vi "Table Control_2D.vi"(0 "CtlRef":refnum<vi>, 5 "CharIn":i16, 7 "VKey":T1, 9 "ScanCode":i16) -> (6 "CharOut":i16, 15 "Discard?":bool)   [LabVIEW 2013]
uses:
  <vilib>/Utility/miscctls.llb/LVRowAndColumnTypeDef.ctl
  <vilib>/event_ctls.llb/eventvkey.ctl
panel:
  in  "Header Row(F)/Column(T)":bool
  in  "Valid Indexes":i32[](array[numeric])
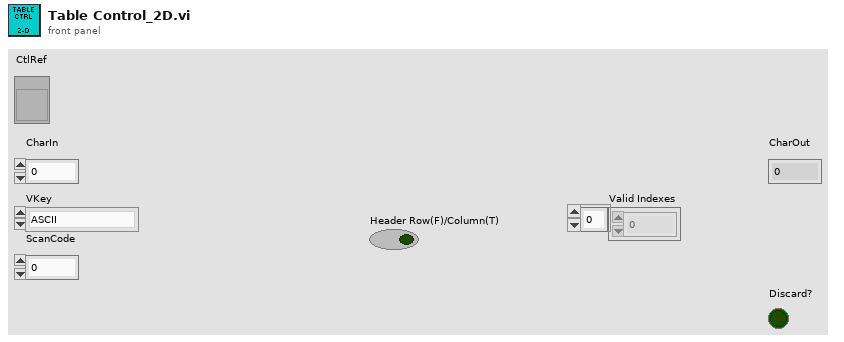
[diagram p1: front panel]
types:
  T1 = typedef "eventvkey.ctl" = enum16{"ASCII", "Enter", "Return", "Shift", "Ctrl", "Alt", "Cmd", "Opt", "Caps", "NumLock", "Clear", "Break", "Up", "Down", "Left", "Right", "Insert", "Delete", "Home", "End", "PageUp", "PageDown", "Escape", "Help", "Pause", "ScrollLock", "F1", "F2", "F3", "F4", "F5", "F6", "F7", "F8", "F9", "F10", "F11", "F12", "F13", "F14", "F15", "F16", "F17", "F18", "F19", "F20", "F21", "F22", "F23", "F24", "Play", "VolumeUp", "VolumeDown", "Mute", "Two Byte Char"}
  T2 = typedef "LVRowAndColumnTypeDef.ctl" = cluster{"Row":i32, "Column":i32}
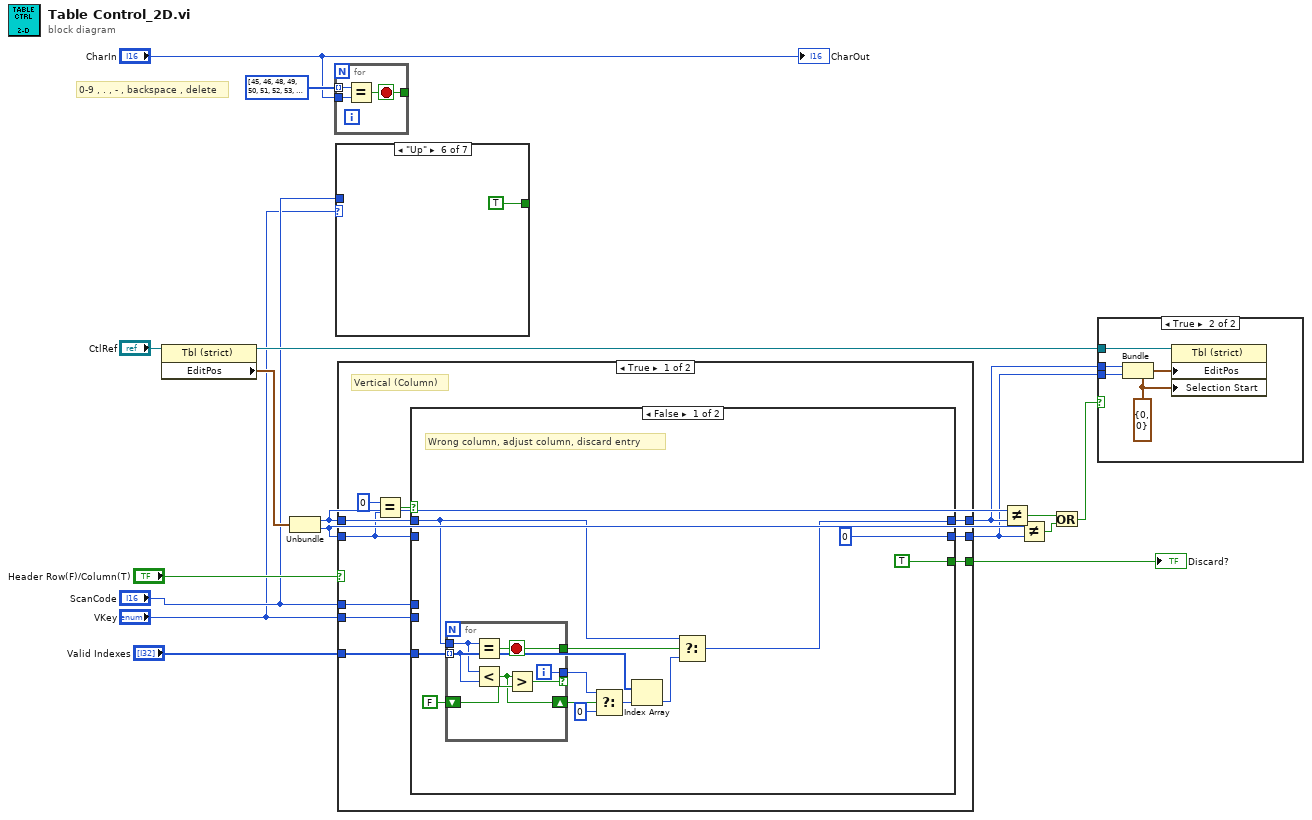
[diagram p0: block diagram]
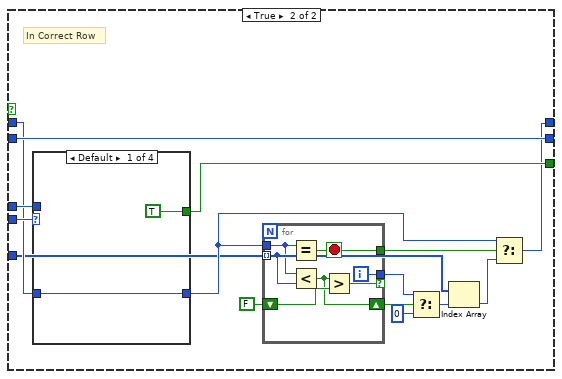
[diagram p3: hidden frame]
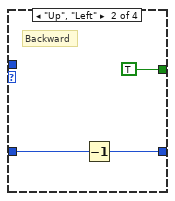
[diagram p4: hidden frame]
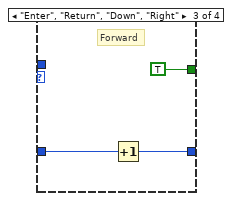
[diagram p5: hidden frame]
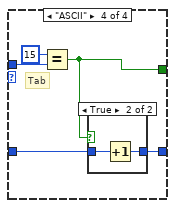
[diagram p6: hidden frame]
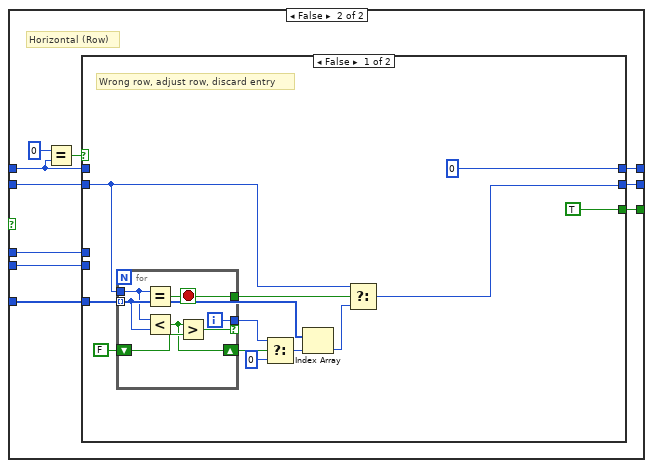
[diagram p8: hidden frame]
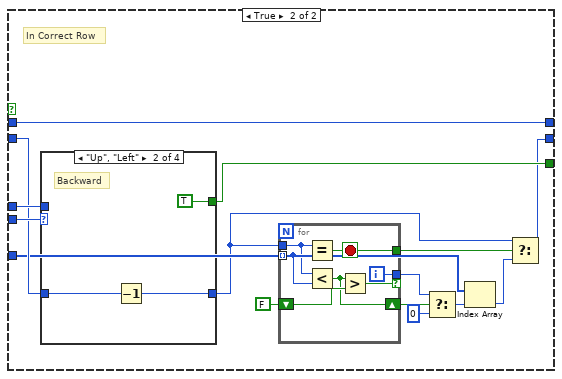
[diagram p9: hidden frame]
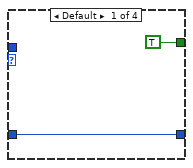
[diagram p10: hidden frame]
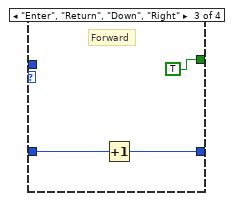
[diagram p11: hidden frame]
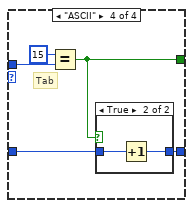
[diagram p12: hidden frame]
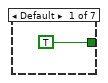
[diagram p14: hidden frame]
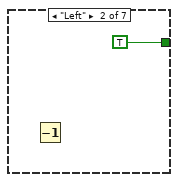
[diagram p15: hidden frame]
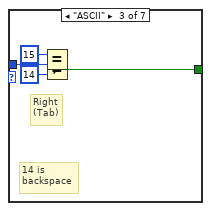
[diagram p16: hidden frame]
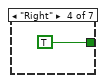
[diagram p17: hidden frame]
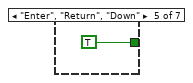
[diagram p18: hidden frame]
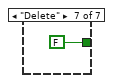
[diagram p19: hidden frame]
diagram:
  # "0-9 , . , - , backspace , delete"
  n1 = property on="Property Node" class="Tbl (strict)"(reference="CtlRef") -> (reference out=w4:refnum<vi>, "EditPos"=w5:T2)  [unwired: 1 in, 1 out]
  n2 = Unbundle(w5) -> ("Row"=w11:i32, "Column"=w9:i32)
  n3 = for {
    tunnel: i16[] [45, 46, 48, 49, 50, 51, 52, 53, 54, 55, 56, 57] -> [w20] mode=indexing
    tunnel: "CharIn" -> [w19]
    tunnel: [w18] -> _
    stop <- w18 stop-if-true
    n4 = Equal?(x=w20, y=w19) -> (x = y?=w18:bool)
  }
  n5 = case shown="\"Up\"" "VKey" {
    tunnel: "ScanCode" -> [_ _ w27 _ _ _ _]
    tunnel: [TRUE TRUE w25 TRUE TRUE TRUE FALSE] -> _
    frame Default {
    }
    frame "Left" {
      n6 = Decrement() -> (x=w24:dbl, x-1=w23:dbl)
    }
    frame "ASCII" {
      # "14 is\nbackspace"
      # "Right\n(Tab)"
      n7 = Equal?(x=i16 15, y=w27) -> ()  [unwired: 1 out]
      n8 = Not Equal?(x=w27, y=i16 14 ("x")) -> (x != y?=w25:bool)
    }
    frame "Right" {
    }
    frame "Enter", "Return", "Down" {
    }
    frame "Up" {
    }
    frame "Delete" {
    }
  }
  n9 = case shown="True" "Header Row(F)/Column(T)" {
    tunnel: w11 -> [w42 w103]
    tunnel: w9 -> [w34 w107]
    tunnel: "Valid Indexes" -> [w36 w106]
    tunnel: [w41 w105] -> w10
    tunnel: [w40 w104] -> w8
    tunnel: [w39 w102] -> w1
    tunnel: "ScanCode" -> [w38 w101]
    tunnel: "VKey" -> [w37 w100]
    frame True {
      # "Vertical (Column)"
      n10 = Equal?(x=0, y=w34) -> (x = y?=w33:bool)
      n11 = case shown="False" w33 {
        tunnel: w34 -> [_ w73]
        tunnel: w36 -> [w48 w62]
        tunnel: [w44 w63] -> w41
        tunnel: [0 w73] -> w40
        tunnel: w42 -> [w45 w72]
        tunnel: [TRUE w74] -> w39
        tunnel: w38 -> [_ w76]
        tunnel: w37 -> [_ w75]
        frame False {
          # "Wrong column, adjust column, discard entry"
          n12 = for {
            tunnel: w48 -> [w59] mode=indexing
            tunnel: w45 -> [w60]
            tunnel: [w61] -> w54
            shift-right: [w55] -> w52
            shift-left: FALSE -> [w58]
            tunnel: [w57] -> w51 if=w56
            i -> [w57]
            stop <- w61 stop-if-true
            n13 = Equal?(x=w60, y=w59) -> (x = y?=w61:bool)
            n14 = Less?(x=w60, y=w59) -> (x < y?=w55:bool)
            n15 = Greater?(x=w55, y=w58) -> (0:w56:bool)
          }
          n16 = Select(t=w51, s=w52, f=0) -> (s? t:f=w49:i32)
          n17 = Index Array(array=w48, index=w49) -> (element=w47:i32)
          n18 = Select(t=w45, s=w54, f=w47) -> (s? t:f=w44:i32)
        }
        frame True {
          # "In Correct Row"
          n19 = case shown="Default" w75 {
            tunnel: w76 -> [_ _ _ w95]
            tunnel: w72 -> [w85 w87 w90 w94]
            tunnel: [w85 w86 w89 w93] -> w64
            tunnel: [TRUE TRUE TRUE w92] -> w74
            frame Default {
            }
            frame "Up", "Left" {
              # "Backward"
              n20 = Decrement(x=w87) -> (x-1=w86:i32)
            }
            frame "Enter", "Return", "Down", "Right" {
              # "Forward"
              n21 = Increment(x=w90) -> (x+1=w89:i32)
            }
            frame "ASCII" {
              # "Tab"
              n22 = Equal?(x=i16 15, y=w95) -> (x = y?=w92:bool)
              n23 = case shown="True" w92 {
                tunnel: w94 -> [w97 w99]
                tunnel: [w97 w98] -> w93
                frame False {
                }
                frame True {
                  n24 = Increment(x=w99) -> (x+1=w98:i32)
                }
              }
            }
          }
          n25 = for {
            tunnel: w62 -> [w81] mode=indexing
            tunnel: w64 -> [w82]
            tunnel: [w83] -> w71
            shift-right: [w77] -> w69
            shift-left: FALSE -> [w80]
            tunnel: [w79] -> w68 if=w78
            i -> [w79]
            stop <- w83 stop-if-true
            n26 = Equal?(x=w82, y=w81) -> (x = y?=w83:bool)
            n27 = Less?(x=w82, y=w81) -> (x < y?=w77:bool)
            n28 = Greater?(x=w77, y=w80) -> (0:w78:bool)
          }
          n29 = Select(t=w68, s=w69, f=0) -> (s? t:f=w66:i32)
          n30 = Index Array(array=w62, index=w66) -> (element=w65:i32)
          n31 = Select(t=w64, s=w71, f=w65) -> (s? t:f=w63:i32)
        }
      }
    }
    frame False {
      # "Horizontal (Row)"
      n32 = Equal?(x=0, y=w103) -> (x = y?=w108:bool)
      n33 = case shown="False" w108 {
        tunnel: w107 -> [w112 w140]
        tunnel: w106 -> [w114 w130]
        tunnel: [0 w143] -> w105
        tunnel: [w111 w131] -> w104
        tunnel: w103 -> [_ w143]
        tunnel: [TRUE w139] -> w102
        tunnel: w101 -> [_ w142]
        tunnel: w100 -> [_ w141]
        frame False {
          # "Wrong row, adjust row, discard entry"
          n34 = for {
            tunnel: w114 -> [w126] mode=indexing
            tunnel: w112 -> [w127]
            tunnel: [w128] -> w120
            shift-right: [w122] -> w118
            shift-left: FALSE -> [w125]
            tunnel: [w124] -> w117 if=w123
            i -> [w124]
            stop <- w128 stop-if-true
            n35 = Equal?(x=w127, y=w126) -> (x = y?=w128:bool)
            n36 = Less?(x=w127, y=w126) -> (x < y?=w122:bool)
            n37 = Greater?(x=w122, y=w125) -> (0:w123:bool)
          }
          n38 = Select(t=w117, s=w118, f=0) -> (s? t:f=w115:i32)
          n39 = Index Array(array=w114, index=w115) -> (element=w113:i32)
          n40 = Select(t=w112, s=w120, f=w113) -> (s? t:f=w111:i32)
        }
        frame True {
          # "In Correct Row"
          n41 = case shown="\"Up\", \"Left\"" w141 {
            tunnel: w142 -> [_ _ _ w162]
            tunnel: w140 -> [w152 w154 w157 w161]
            tunnel: [w152 w153 w156 w160] -> w129
            tunnel: [TRUE TRUE TRUE w159] -> w139
            frame Default {
            }
            frame "Up", "Left" {
              # "Backward"
              n42 = Decrement(x=w154) -> (x-1=w153:i32)
            }
            frame "Enter", "Return", "Down", "Right" {
              # "Forward"
              n43 = Increment(x=w157) -> (x+1=w156:i32)
            }
            frame "ASCII" {
              # "Tab"
              n44 = Equal?(x=i16 15, y=w162) -> (x = y?=w159:bool)
              n45 = case shown="True" w159 {
                tunnel: w161 -> [w164 w166]
                tunnel: [w164 w165] -> w160
                frame False {
                }
                frame True {
                  n46 = Increment(x=w166) -> (x+1=w165:i32)
                }
              }
            }
          }
          n47 = for {
            tunnel: w130 -> [w148] mode=indexing
            tunnel: w129 -> [w149]
            tunnel: [w150] -> w138
            shift-right: [w144] -> w136
            shift-left: FALSE -> [w147]
            tunnel: [w146] -> w135 if=w145
            i -> [w146]
            stop <- w150 stop-if-true
            n48 = Equal?(x=w149, y=w148) -> (x = y?=w150:bool)
            n49 = Less?(x=w149, y=w148) -> (x < y?=w144:bool)
            n50 = Greater?(x=w144, y=w147) -> (0:w145:bool)
          }
          n51 = Select(t=w135, s=w136, f=0) -> (s? t:f=w133:i32)
          n52 = Index Array(array=w130, index=w133) -> (element=w132:i32)
          n53 = Select(t=w129, s=w138, f=w132) -> (s? t:f=w131:i32)
        }
      }
    }
  }
  "Discard?" <- w1
  n54 = Not Equal?(x=w11, y=w10) -> (x != y?=w12:bool)
  n55 = Not Equal?(x=w9, y=w8) -> (x != y?=w13:bool)
  n56 = Or(x=w12, y=w13) -> (x .or. y?=w14:bool)
  n57 = case shown="True" w14 {
    tunnel: w4 -> [_ w171]
    tunnel: w8 -> [_ w168]
    tunnel: w10 -> [_ w167]
    frame False {
    }
    frame True {
      w169 = T2 {"Row"=0, "Column"=0} ("Active Cell:Active Cell")
      n58 = Bundle(cluster=w169, "Row"=w167, "Column"=w168) -> (w170:T2)
      n59 = property on="Property Node" class="Tbl (strict)"(reference=w171, "EditPos"=w170, "Selection Start"=w169) -> ()  [unwired: 1 in, 2 out]
    }
  }
  "CharOut" <- "CharIn"
